vi "AcquireContinuous.vi"(8 "error in (no error)":errorcluster, 9 "frames number":i32, 10 "exp_time":u16=100, 11 "hCam":i16) -> (0 "error out":errorcluster, 3 "frame data":dbl[][](array[numeric]))   [LabVIEW 2021]
uses:
  src/Low_level_subVIs/PVCAM_rgn_type.ctl
  LabVIEW.exe
panel:
  in  "stop":bool
  out "Intensity Graph":dbl[][](graph)
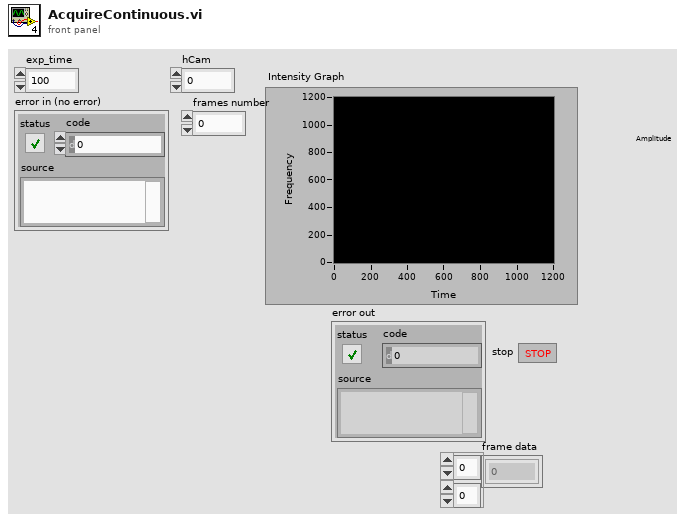
[diagram p1: front panel]
types:
  T1 = enum16{"CCS_NO_CHANGE", "CCS_HALT", "CCS_HALT_CLOSE_SHTR", "CCS_CLEAR", "CCS_CLEAR_CLOSE_SHTR", "CCS_OPEN_SHTR", "CCS_CLEAR_OPEN_SHTR"}
  T2 = enum16{"CIRC_NONE", "CIRC_OVERWRITE", "CIRC_NO_OVERWRITE"}
  T3 = typedef "PVCAM_rgn_type.ctl" = cluster{"s1":u16, "s2":u16, "sbin":u16, "p1":u16, "p2":u16, "pbin":u16}
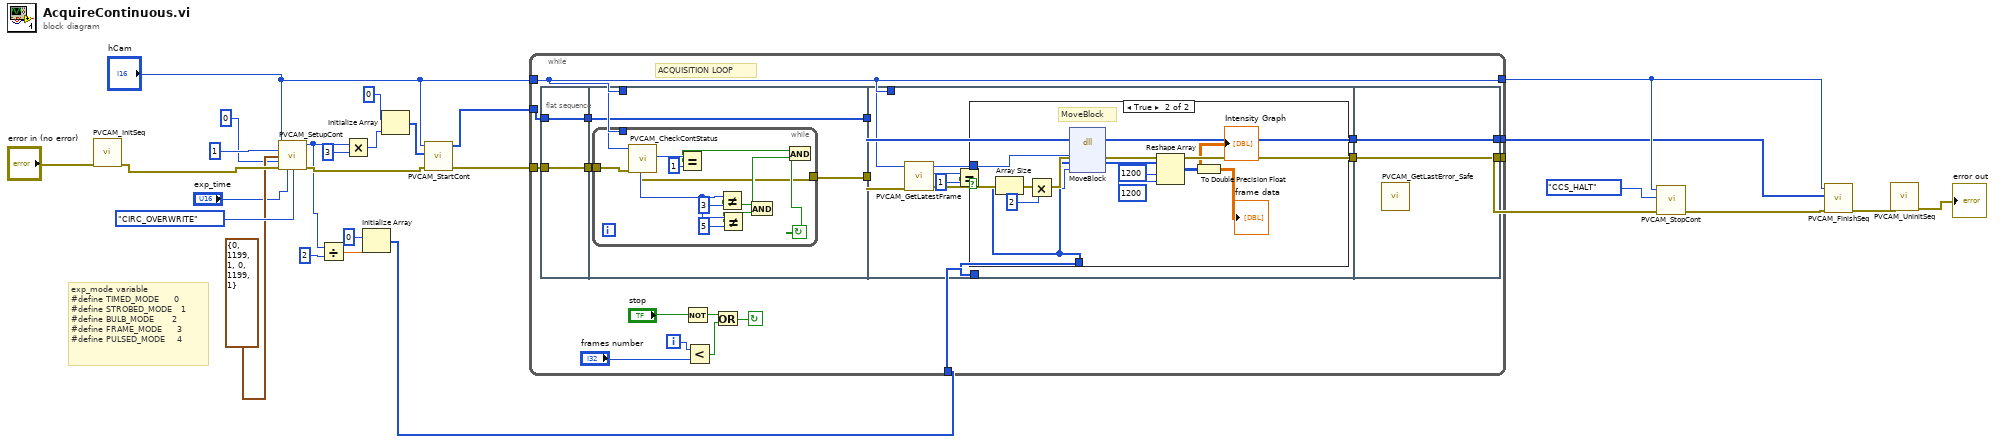
[diagram p0: block diagram]
diagram:
  # "exp_mode variable\n#define TIMED_MODE     0\n#define STROBED_MODE   1\n#define BULB_MODE      2\n#define FRAME_MODE     3\n#define PULSED_MODE    4"
  n1 = call "PVCAM_InitSeq.vi"("error in (no error)"="error in (no error)") -> ("error out"=w26:errorcluster)  [unwired: 9 in, 1 out]
  n2 = call "PVCAM_SetupCont.vi"("hCam"="hCam", "rgn_total"=u16 1 ("exp_total"), "rgn_type"=T3 {"s1"=0, "s2"=1199, "sbin"=1, "p1"=0, "p2"=1199, "pbin"=1}, "exp_mode"=i16 0, "error in (no error)"=w26, "exp_time"="exp_time", "circ_mode"=T2."CIRC_OVERWRITE") -> ("stream_size"=w3:u32, "error out"=w19:errorcluster)  [unwired: 6 in, 1 out]
  n3 = Divide(x=w3, y=u32 2) -> (x/y=w1:dbl)
  n4 = Multiply(x=w3, y=u32 3) -> (x*y=w21:u32)
  n5 = Initialize Array(u16 0 ("element"), w1) -> (w6:u16[])
  n6 = Initialize Array(u16 0 ("element"), w21) -> (w20:u16[])
  n7 = call "PVCAM_StartCont.vi"("error in (no error)"=w19, "buffer"=w20, "hCam"="hCam") -> ("error out"=w16:errorcluster, "ImageBuf"=w9:u8[])  [unwired: 6 in, 1 out]
  n8 = while {
    tunnel: "hCam" -> [w38]
    tunnel: w16 -> [w44]
    tunnel: [w40] -> w10
    tunnel: [w38] -> w12
    tunnel: w9 -> [w42]
    tunnel: [w39] -> w8
    tunnel: w6 -> [w37]
    i -> [w45]
    stop <- w31 continue-if-true
    # "ACQUISITION LOOP"
    n9 = flat-sequence {
      tunnel: w42 -> [w46]
      tunnel: w44 -> [w47]
      tunnel: [w47] -> w34
      tunnel: [w46] -> w33
      tunnel: w38 -> [w50]
      tunnel: [w49] -> w43
      tunnel: [w48] -> w41
      tunnel: w34 -> [w51]
      tunnel: w33 -> [w48]
      tunnel: w43 -> [w73]
      tunnel: w41 -> [w71]
      tunnel: w38 -> [w70]
      tunnel: w37 -> [w68]
      tunnel: [w72] -> w36
      tunnel: [w71] -> w35
      tunnel: [w84] -> w39
      tunnel: [w85] -> w40
      tunnel: w36 -> [w85]
      tunnel: w35 -> [w84]
      frame #0 {
      }
      frame #1 {
        n10 = while {
          tunnel: w50 -> [w64]
          tunnel: [w53] -> w49
          tunnel: w51 -> [w52]
          stop <- w54 continue-if-true
          n11 = call "PVCAM_CheckContStatus.vi"("error in (no error)"=w52, "hCam"=w64) -> ("error out"=w53:errorcluster, "return type"=w60:i16, "status"=w62:i16)  [unwired: 5 in, 2 out]
          n12 = Equal?(x=w60, y=i16 1) -> (x = y?=w58:bool)
          n13 = Not Equal?(x=w62, y=i16 3) -> (x != y?=w57:bool)
          n14 = Not Equal?(x=w62, y=i16 5) -> (x != y?=w56:bool)
          n15 = And(x=w57, y=w56) -> (x .and. y?=w55:bool)
          n16 = And(x=w58, y=w55) -> (x .and. y?=w54:bool)
        }
      }
      frame #2 {
        n17 = call "PVCAM_GetLatestFrame.vi"("error in (no error)"=w73, "hCam"=w70) -> ("error out"=w72:errorcluster, "return"=w67:i16, "frame ptr"=w69:u64)  [unwired: 6 in]
        n18 = Equal?(x=w67, y=i16 1) -> (x = y?=w65:bool)
        n19 = case shown="True" w65 {
          tunnel: w69 -> [_ w79]
          tunnel: w68 -> [_ w78]
          frame False {
          }
          frame True {
            # "MoveBlock"
            n20 = Array Size(array=w78) -> (size(s)=w76:i32)
            n21 = Multiply(x=w76, y=2) -> (x*y=w74:i32)
            n22 = dll-call lib="LabVIEW.exe" fn="MoveBlock"("source"=w79, "dest"=w78, "size"=w74) -> ("dest"=w77:u16[])  [unwired: 6 in, 2 out]
            n23 = Reshape Array(w77, 1200 ("dimension size"), 1200 ("dimension size")) -> (w82:u16[][])
            n24 = To Double Precision Float(number=w82) -> (double precision float=→"Intensity Graph" →"frame data":dbl[][])
          }
        }
      }
      frame #3 {
        n25 = call "PVCAM_GetLastError_Safe.vi"() -> ()  [unwired: 11 in, 1 out]
      }
    }
    n26 = Not(x="stop") -> (.not. x?=w29:bool)
    n27 = Less?(x=w45, y="frames number") -> (x < y?=w30:bool)
    n28 = Or(x=w29, y=w30) -> (x .or. y?=w31:bool)
  }
  n29 = call "PVCAM_StopCont.vi"("error in (no error)"=w10, "cam_state"=T1."CCS_HALT", "hCam"=w12) -> ("error out"=w11:errorcluster)  [unwired: 7 in, 1 out]
  n30 = call "PVCAM_FinishSeq.vi"("error in (no error)"=w11, "buffer"=w8, "hCam"=w12) -> ("error out"=w14:errorcluster)  [unwired: 7 in, 1 out]
  n31 = call "PVCAM_UninitSeq.vi"("error in (no error)"=w14) -> ("error out"=→"error out":errorcluster)  [unwired: 9 in, 1 out]
